vi "MGCC_FntStaMach_Manual panel.vi"(1 "current state":string) -> (0 "event":bool[](array[boolean]))   [LabVIEW 2016]
doc: "-----------------------------------------------------------------------------------------------------------------------\nCopyright <2019> <The University of Tennessee at Knoxville and the University of Tennessee Research Foundation>\nThis software is released under BSD-3 \nhttps://opensource.org/licenses/BSD-3-Clause \nAdditional license options available at https://utrf.tennessee.edu/industry/sample-agreements/\n-----------------------------------------------------------------------------------------------------------------------"
panel:
  in  "OFF":bool
  in  "STD":bool
  in  "ABN":bool
  in  "FLT":bool
  in  "FLT":bool
  in  "ABN":bool
  in  "BKS":bool
  in  "I2G":bool
  in  "STD":bool
  in  "G2I_IN":bool
  in  "G2I_UN":bool
  in  "ISD":bool
  in  "GC":bool
  in  "ISD":bool
  in  "FLT":bool
  in  "ABN":bool
  in  "BKS":bool
  in  "STD":bool
  in  "GC":bool
  in  "FLT":bool
  in  "ABN":bool
  in  "I2G":bool
  in  "STD":bool
  in  "G2I_IN":bool
  in  "FLT":bool
  in  "ABN":bool
  in  "ISD":bool
  in  "STD":bool
  in  "G2I_UN":bool
  in  "FLT":bool
  in  "ABN":bool
  in  "ISD":bool
  in  "STD":bool
  in  "FLT":bool
  in  "ABN":bool
  in  "ISD":bool
  in  "I2G":bool
  in  "FLT":bool
  in  "ABN":bool
  in  "G2I_IN":bool
  in  "G2I_UN":bool
  in  "GC":bool
  in  "FLT":bool
  in  "ABN":bool
  in  "STD":bool
  in  "BKS":bool
  in  "ISD":bool
  in  "GC":bool
  in  "STD":bool
  in  "ABN":bool
  in  "FLT":bool
  # "OFF State"
  # "STD State"
  # "GC State"
  # "BKS State"
  # "ISD State"
  # "ABN State"
  # "G2I_UN State"
  # "G2I_IN State"
  # "FLT State"
  # "I2G State"
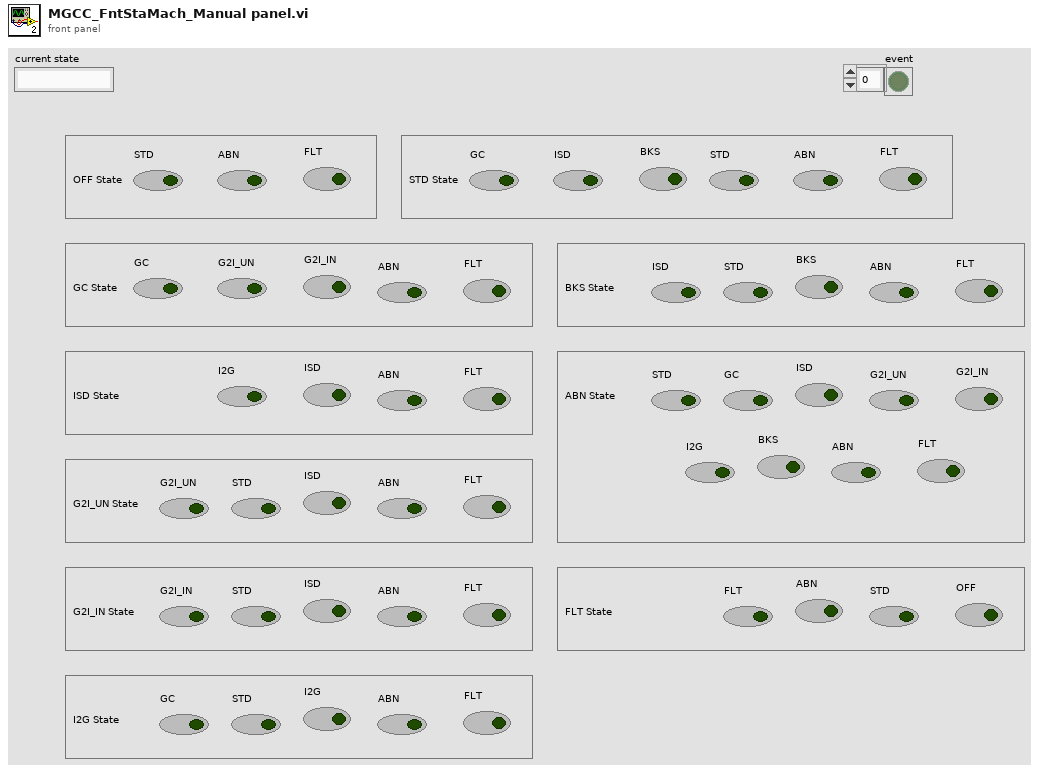
[diagram p1: front panel]
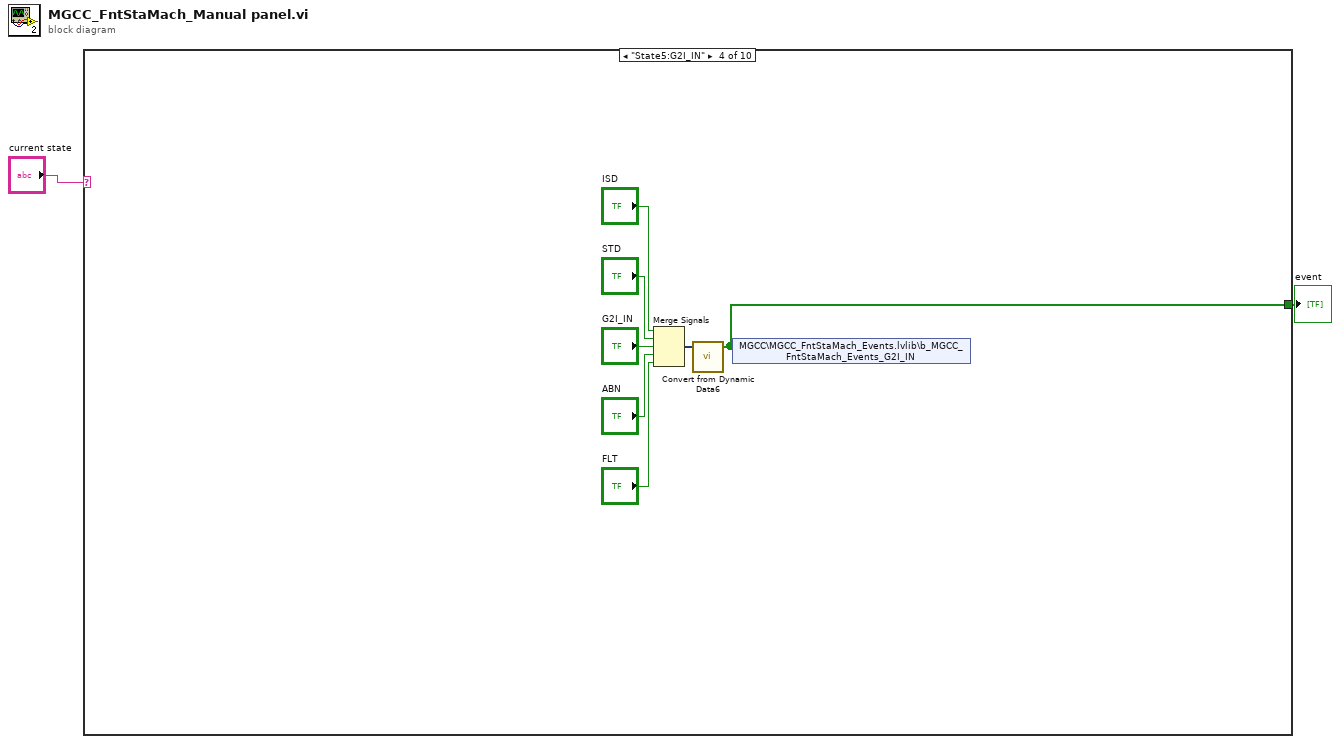
[diagram p0: block diagram]
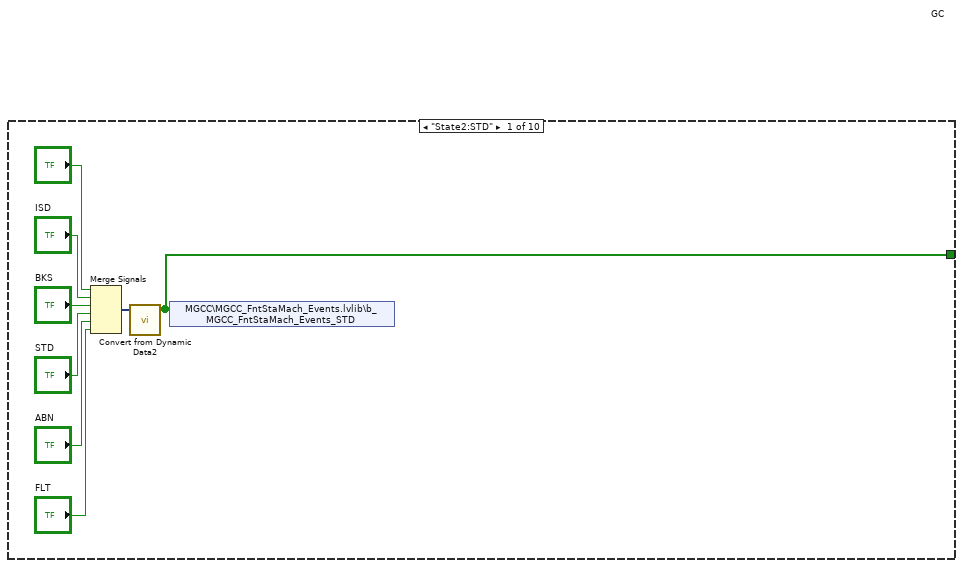
[diagram p2: hidden frame]
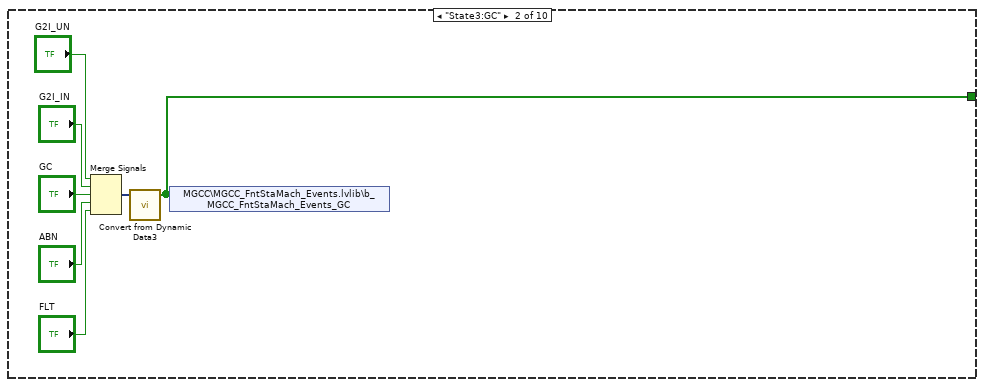
[diagram p3: hidden frame]
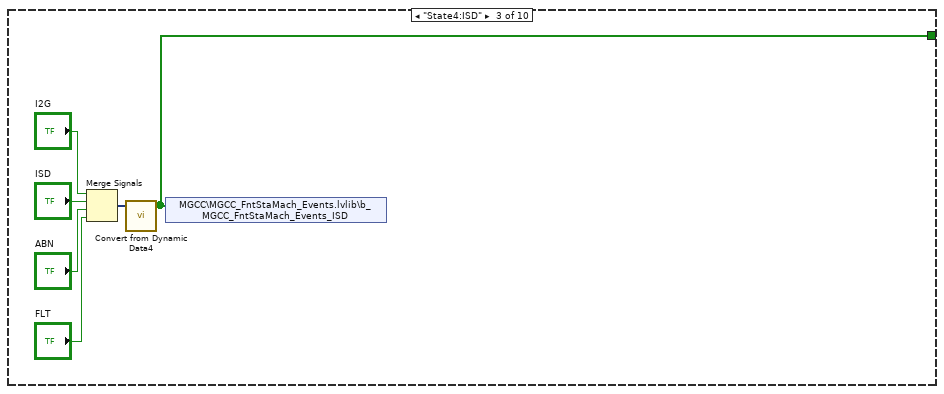
[diagram p4: hidden frame]
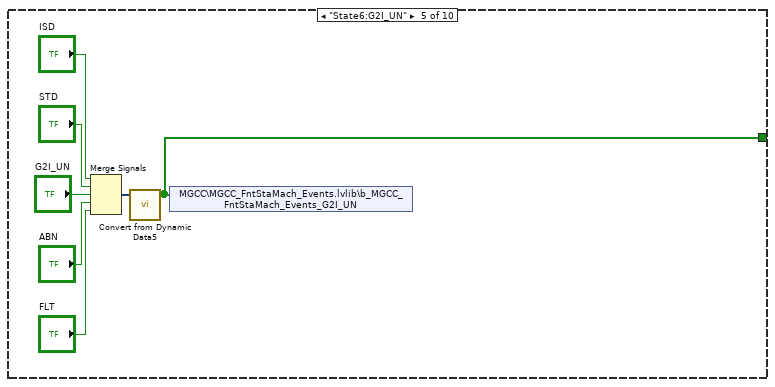
[diagram p5: hidden frame]
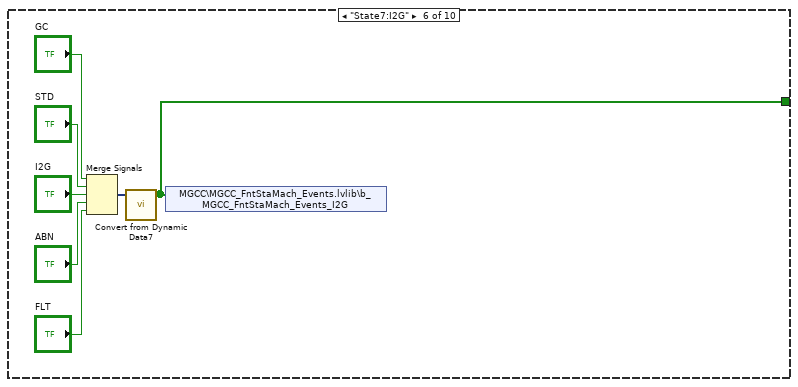
[diagram p6: hidden frame]
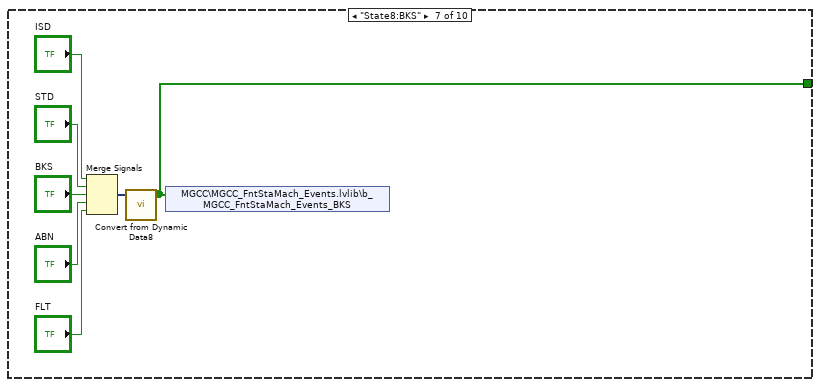
[diagram p7: hidden frame]
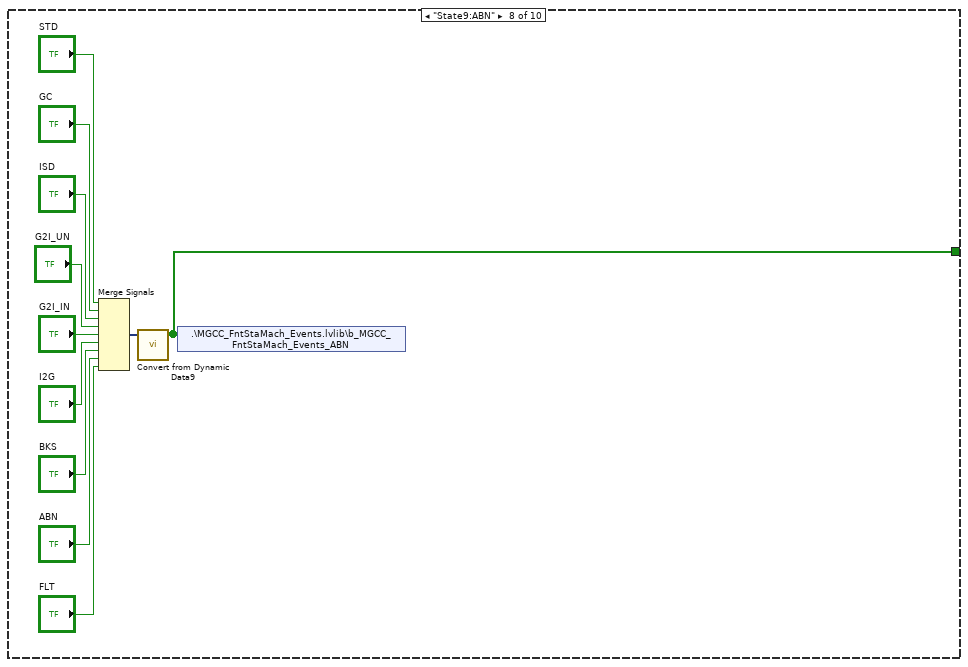
[diagram p8: hidden frame]
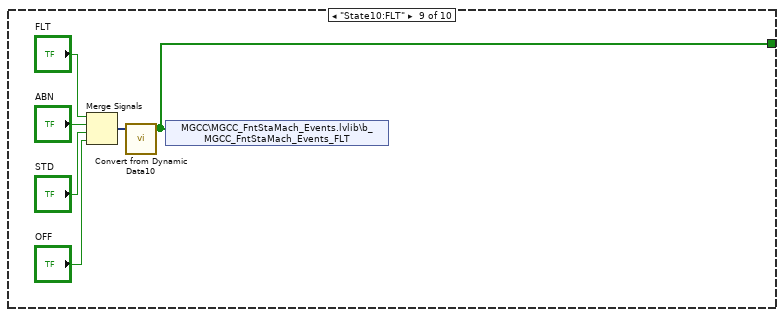
[diagram p9: hidden frame]
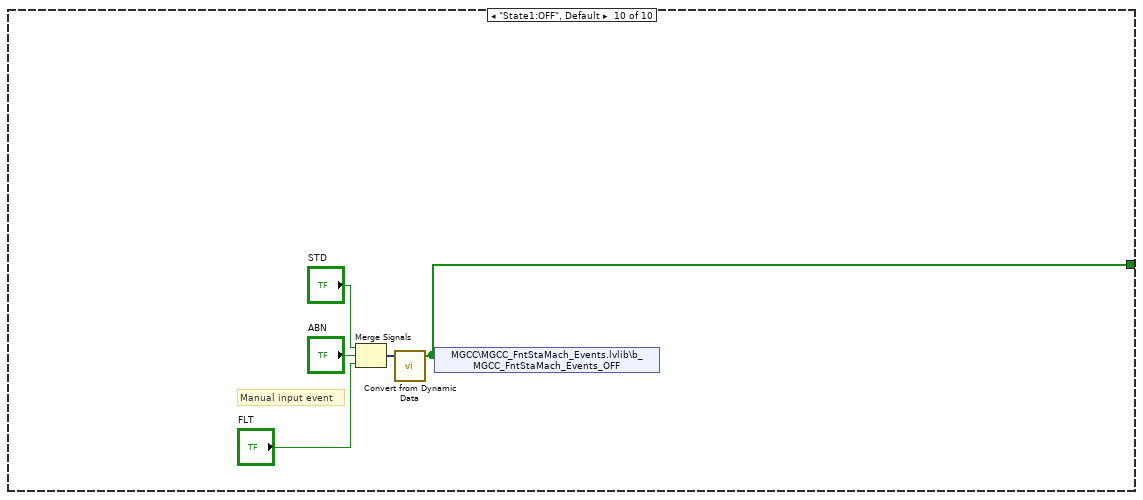
[diagram p10: hidden frame]
diagram:
  n1 = case shown="\"State5:G2I_IN\"" "current state" {
    tunnel: [w3 w11 w18 w24 w31 w38 w45 w52 w63 w69] -> w1
    frame "State2:STD" {
      n2 = Merge Signals("GC", "ISD", "BKS", "STD", "ABN", "FLT") -> (w4:dynamicdata)
      n3 = call "Convert from Dynamic Data2"("Dynamic Data Type"=w4) -> ("Array"=w3:bool[])  [unwired: 3 in]
      n4 = shared-variable "MGCC\\MGCC_FntStaMach_Events.lvlib\\b_MGCC_FntStaMach_Events_STD"(w3) -> ()  [unwired: 1 in, 1 out]
    }
    frame "State3:GC" {
      n5 = Merge Signals("G2I_UN", "G2I_IN", "GC", "ABN", "FLT") -> (w12:dynamicdata)
      n6 = call "Convert from Dynamic Data3"("Dynamic Data Type"=w12) -> ("Array"=w11:bool[])  [unwired: 3 in]
      n7 = shared-variable "MGCC\\MGCC_FntStaMach_Events.lvlib\\b_MGCC_FntStaMach_Events_GC"(w11) -> ()  [unwired: 1 in, 1 out]
    }
    frame "State4:ISD" {
      n8 = Merge Signals("I2G", "ISD", "ABN", "FLT") -> (w19:dynamicdata)
      n9 = call "Convert from Dynamic Data4"("Dynamic Data Type"=w19) -> ("Array"=w18:bool[])  [unwired: 3 in]
      n10 = shared-variable "MGCC\\MGCC_FntStaMach_Events.lvlib\\b_MGCC_FntStaMach_Events_ISD"(w18) -> ()  [unwired: 1 in, 1 out]
    }
    frame "State5:G2I_IN" {
      n11 = Merge Signals("ISD", "STD", "G2I_IN", "ABN", "FLT") -> (w25:dynamicdata)
      n12 = call "Convert from Dynamic Data6"("Dynamic Data Type"=w25) -> ("Array"=w24:bool[])  [unwired: 3 in]
      n13 = shared-variable "MGCC\\MGCC_FntStaMach_Events.lvlib\\b_MGCC_FntStaMach_Events_G2I_IN"(w24) -> ()  [unwired: 1 in, 1 out]
    }
    frame "State6:G2I_UN" {
      n14 = Merge Signals("ISD", "STD", "G2I_UN", "ABN", "FLT") -> (w32:dynamicdata)
      n15 = call "Convert from Dynamic Data5"("Dynamic Data Type"=w32) -> ("Array"=w31:bool[])  [unwired: 3 in]
      n16 = shared-variable "MGCC\\MGCC_FntStaMach_Events.lvlib\\b_MGCC_FntStaMach_Events_G2I_UN"(w31) -> ()  [unwired: 1 in, 1 out]
    }
    frame "State7:I2G" {
      n17 = Merge Signals("GC", "STD", "I2G", "ABN", "FLT") -> (w39:dynamicdata)
      n18 = call "Convert from Dynamic Data7"("Dynamic Data Type"=w39) -> ("Array"=w38:bool[])  [unwired: 3 in]
      n19 = shared-variable "MGCC\\MGCC_FntStaMach_Events.lvlib\\b_MGCC_FntStaMach_Events_I2G"(w38) -> ()  [unwired: 1 in, 1 out]
    }
    frame "State8:BKS" {
      n20 = Merge Signals("ISD", "STD", "BKS", "ABN", "FLT") -> (w46:dynamicdata)
      n21 = call "Convert from Dynamic Data8"("Dynamic Data Type"=w46) -> ("Array"=w45:bool[])  [unwired: 3 in]
      n22 = shared-variable "MGCC\\MGCC_FntStaMach_Events.lvlib\\b_MGCC_FntStaMach_Events_BKS"(w45) -> ()  [unwired: 1 in, 1 out]
    }
    frame "State9:ABN" {
      n23 = Merge Signals("STD", "GC", "ISD", "G2I_UN", "G2I_IN", "I2G", "BKS", "ABN", "FLT") -> (w53:dynamicdata)
      n24 = call "Convert from Dynamic Data9"("Dynamic Data Type"=w53) -> ("Array"=w52:bool[])  [unwired: 3 in]
      n25 = shared-variable ".\\MGCC_FntStaMach_Events.lvlib\\b_MGCC_FntStaMach_Events_ABN"(w52) -> ()  [unwired: 1 in, 1 out]
    }
    frame "State10:FLT" {
      n26 = Merge Signals("FLT", "ABN", "STD", "OFF") -> (w64:dynamicdata)
      n27 = call "Convert from Dynamic Data10"("Dynamic Data Type"=w64) -> ("Array"=w63:bool[])  [unwired: 3 in]
      n28 = shared-variable "MGCC\\MGCC_FntStaMach_Events.lvlib\\b_MGCC_FntStaMach_Events_FLT"(w63) -> ()  [unwired: 1 in, 1 out]
    }
    frame "State1:OFF", Default {
      # "Manual input event"
      n29 = Merge Signals("STD", "ABN", "FLT") -> (w70:dynamicdata)
      n30 = call "Convert from Dynamic Data"("Dynamic Data Type"=w70) -> ("Array"=w69:bool[])  [unwired: 3 in]
      n31 = shared-variable "MGCC\\MGCC_FntStaMach_Events.lvlib\\b_MGCC_FntStaMach_Events_OFF"(w69) -> ()  [unwired: 1 in, 1 out]
    }
  }
  "event" <- w1
